vi "BuildModule2 (SubVI).vi"(0 "Module side length [mm]":dbl=97.54, 1 "Angle":dbl, 2 "Centre [mm]":cluster{"X":dbl, "Y":dbl, "Z":dbl}, 3 "x to fiducial [um]":dbl=230.0, 4 "y to fiducial [um]":dbl=1030.0, 5 "Units":enum16{"mrad", "Radians", "Degrees"}(ring)) -> (7 "Generated List of Module Coordinates":dbl[][](array[numeric]))   [LabVIEW 2016]
panel:
  in  "stop":bool
  out "Created Module Graph":cluster{dbl[], dbl[]}(graph)
  out "Z":dbl
  out "y+lv":dbl
  out "y-lv":dbl
  out "x-lh":dbl
  out "x+lh":dbl
  out "A [mm]":cluster{"X":dbl, "Y":dbl, "Z":dbl}
  out "D [mm]":cluster{"X":dbl, "Y":dbl, "Z":dbl}
  out "C [mm]":cluster{"X":dbl, "Y":dbl, "Z":dbl}
  out "B [mm]":cluster{"X":dbl, "Y":dbl, "Z":dbl}
  out "lv [mm]":dbl
  out "lh [mm]":dbl
  # "This SubVI takes a centre coordinate and computes the positions of modules associated with that centre.\nThe SubVI also accepts a rotation angle to pivot the module position"
  # "230 um for 4dots"
  # "230+300+500 um for 4dots"
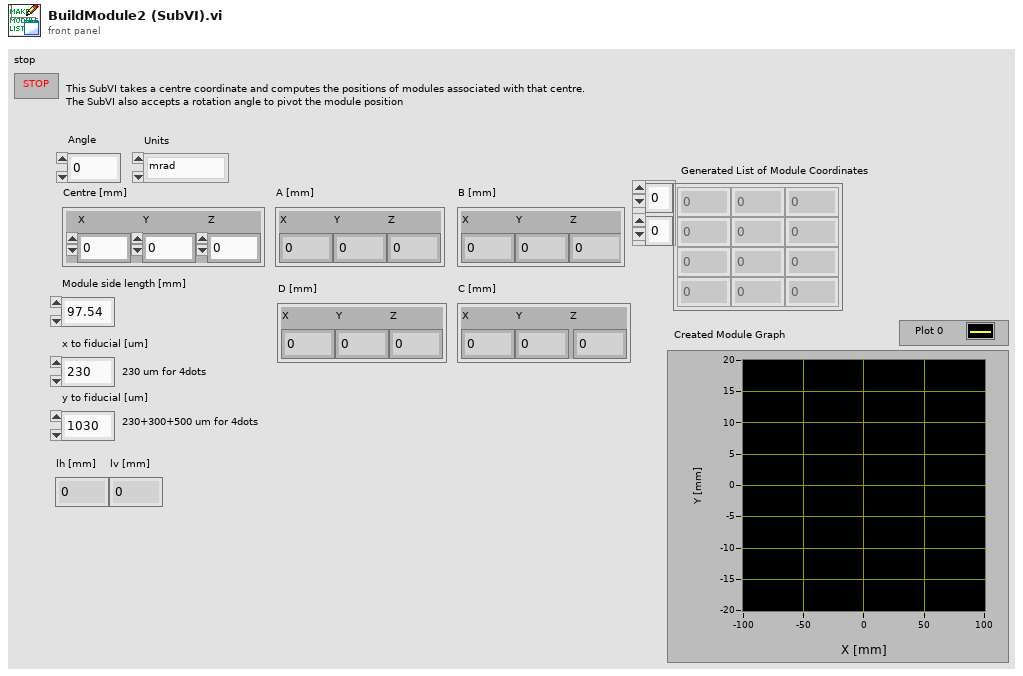
[diagram p1: front panel]
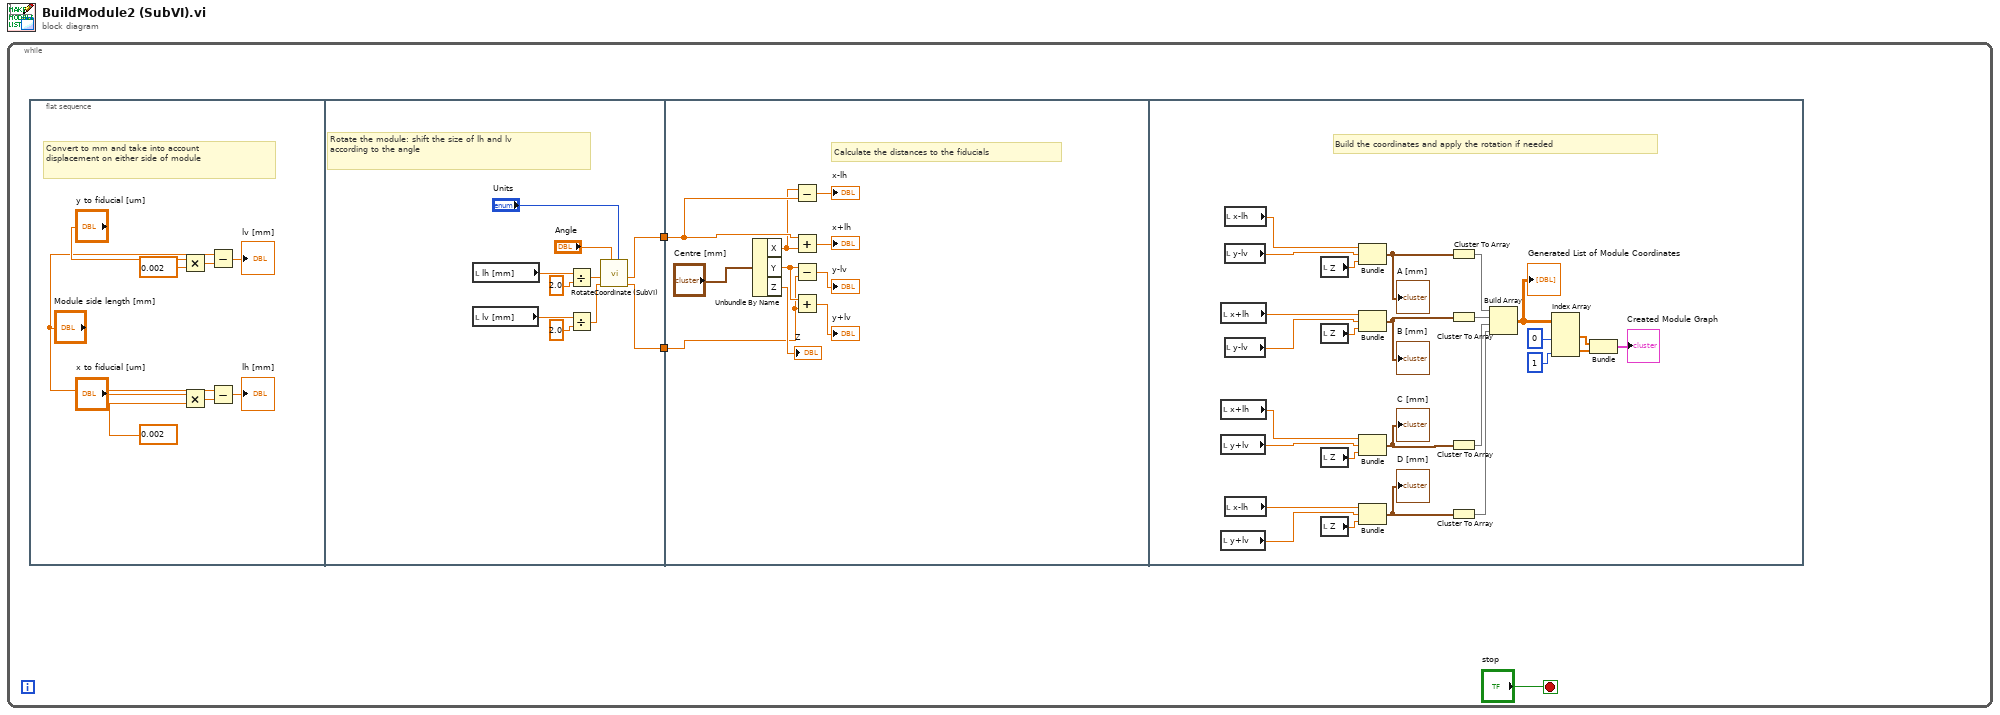
[diagram p0: block diagram]
diagram:
  n1 = while {
    stop <- "stop" stop-if-true
    n2 = flat-sequence {
      tunnel: [w14] -> w2
      tunnel: [w13] -> w1
      tunnel: w2 -> [w26]
      tunnel: w1 -> [w23]
      frame #0 {
        # "Convert to mm and take into account\ndisplacement on either side of module"
        n3 = Multiply(x="y to fiducial [um]", y=0.002) -> (x*y=w5:dbl)
        n4 = Multiply(x="x to fiducial [um]", y=0.002) -> (x*y=w8:dbl)
        n5 = Subtract(x="Module side length [mm]", y=w5) -> (x-y=→"lv [mm]":dbl)
        n6 = Subtract(x="Module side length [mm]", y=w8) -> (x-y=→"lh [mm]":dbl)
      }
      frame #1 {
        # "Rotate the module: shift the size of lh and lv\naccording to the angle"
        n7 = local read "lh [mm]"() -> (w22:dbl)
        n8 = local read "lv [mm]"() -> (w20:dbl)
        n9 = Divide(x=w22, y=2.0) -> (x/y=w18:dbl)
        n10 = Divide(x=w20, y=2.0) -> (x/y=w17:dbl)
        n11 = call "RotateCoordinate (SubVI).vi"("Units"="Units", "Angle"="Angle", "y"=w17, "x"=w18) -> ("y'"=w13:dbl, "x'"=w14:dbl)  [unwired: 6 in]
      }
      frame #2 {
        # "Calculate the distances to the fiducials"
        n12 = Unbundle By Name("Centre [mm]") -> ("X"=w25:dbl, "Y"=w24:dbl, "Z"=→"Z":dbl)
        n13 = Subtract(x=w25, y=w26) -> (x-y=→"x-lh":dbl)
        n14 = Add(x=w26, y=w25) -> (x+y=→"x+lh":dbl)
        n15 = Subtract(x=w24, y=w23) -> (x-y=→"y-lv":dbl)
        n16 = Add(x=w24, y=w23) -> (x+y=→"y+lv":dbl)
      }
      frame #3 {
        # "Build the coordinates and apply the rotation if needed"
        n17 = local read "x+lh"() -> (w52:dbl)
        n18 = local read "x+lh"() -> (w50:dbl)
        n19 = local read "y+lv"() -> (w49:dbl)
        n20 = local read "y+lv"() -> (w46:dbl)
        n21 = local read "x-lh"() -> (w58:dbl)
        n22 = local read "y-lv"() -> (w57:dbl)
        n23 = local read "y-lv"() -> (w53:dbl)
        n24 = local read "x-lh"() -> (w45:dbl)
        n25 = local read "Z"() -> (w56:dbl)
        n26 = local read "Z"() -> (w54:dbl)
        n27 = local read "Z"() -> (w48:dbl)
        n28 = local read "Z"() -> (w47:dbl)
        n29 = Bundle("x-lh"=w58, "y-lv"=w57, "Z"=w56) -> (w55:cluster{"x-lh":dbl, "y-lv":dbl, "Z":dbl})  [unwired: 1 in]
        "A [mm]" <- w55
        n30 = Bundle("x+lh"=w52, "y-lv"=w53, "Z"=w54) -> (w51:cluster{"x+lh":dbl, "y-lv":dbl, "Z":dbl})  [unwired: 1 in]
        "B [mm]" <- w51
        n31 = Bundle("x+lh"=w50, "y+lv"=w49, "Z"=w48) -> (w44:cluster{"x+lh":dbl, "y+lv":dbl, "Z":dbl})  [unwired: 1 in]
        "C [mm]" <- w44
        n32 = Bundle("x-lh"=w45, "y+lv"=w46, "Z"=w47) -> (w43:cluster{"x-lh":dbl, "y+lv":dbl, "Z":dbl})  [unwired: 1 in]
        "D [mm]" <- w43
        n33 = Cluster To Array(cluster=w55) -> (array=w42:dbl[])
        n34 = Cluster To Array(cluster=w51) -> (array=w41:dbl[])
        n35 = Cluster To Array(cluster=w44) -> (array=w40:dbl[])
        n36 = Cluster To Array(cluster=w43) -> (array=w39:dbl[])
        n37 = Build Array(w42, w41, w40, w39) -> (w38:dbl[][])
        "Generated List of Module Coordinates" <- w38
        n38 = Index Array(array=w38, index (col) #1=0 ("disabled index (col)"), index (col) #2=1 ("index (col)")) -> (element #1=w35:dbl[], element #2=w34:dbl[])  [unwired: 2 in]
        n39 = Bundle(w35, w34) -> (→"Created Module Graph":cluster{dbl[], dbl[]})  [unwired: 1 in]
      }
    }
  }
